vi "Host_AutoApproach.vi"() -> ()   [LabVIEW 2014]
uses:
  <vilib>/userdefined/High Color/nirio_resource_hc.ctl
  <vilib>/Instr/_visa.llb/VISA Configure Serial Port (Instr).vi
  <vilib>/FPGAPlugInAG/PCIe-7851R/niLvFpga_Open_PCIe-7851R.vi
  <vilib>/rvi/interface/common/dynamic/niFpgaDynamicAddResources.vi
  <vilib>/Utility/error.llb/Error Cluster From Error Code.vi
  <vilib>/rvi/errors/niLvFpgaAdjustHostInterfaceError.vi
  <vilib>/FPGAPlugInAG/Dynamic/niLvFpga_Run_Dynamic.vi
  <vilib>/FPGAPlugInAG/Dynamic/niLvFpga_Close_Dynamic.vi
  <vilib>/rvi/interface/nirviOpenFPGA/nirviOpenFPGA.xnode
  FPGA Bitfiles/XZFPGAWithinHopp_FPGATarget_ApproachingStep(_Flh4bpoPuwk.lvbitx
  <vilib>/rvi/interface/nirviReadWriteControl/nirviReadWriteControl.xnode
  <vilib>/rvi/interface/nirviMethod/nirviMethod.xnode
  <vilib>/rvi/interface/nirviCloseFPGA/nirviCloseFPGA.xnode
  NiFpgaLv.dll
  <vilib>/rvi/interface/Simulation/niFpgaSimulationCallBeginRW.vi
panel:
  out "ZCalPos":i32
  in  "PIZ":T1
  in  "ContinuousReapproach":bool
  in  "UseMemoryPos?":bool=TRUE
  out "ZRealPos":i16
  out "Curr":i16
  out "PIZPosDia":i16(graph)
  out "CurrDia":i16(graph)
  in  "stop":bool
  out "RoughZPos?":dbl
  out "Error?":string
  in  "RoughZ":refnum<visa-resource-name>
  in  "RoughZInitPos":dbl format="%#_13g"
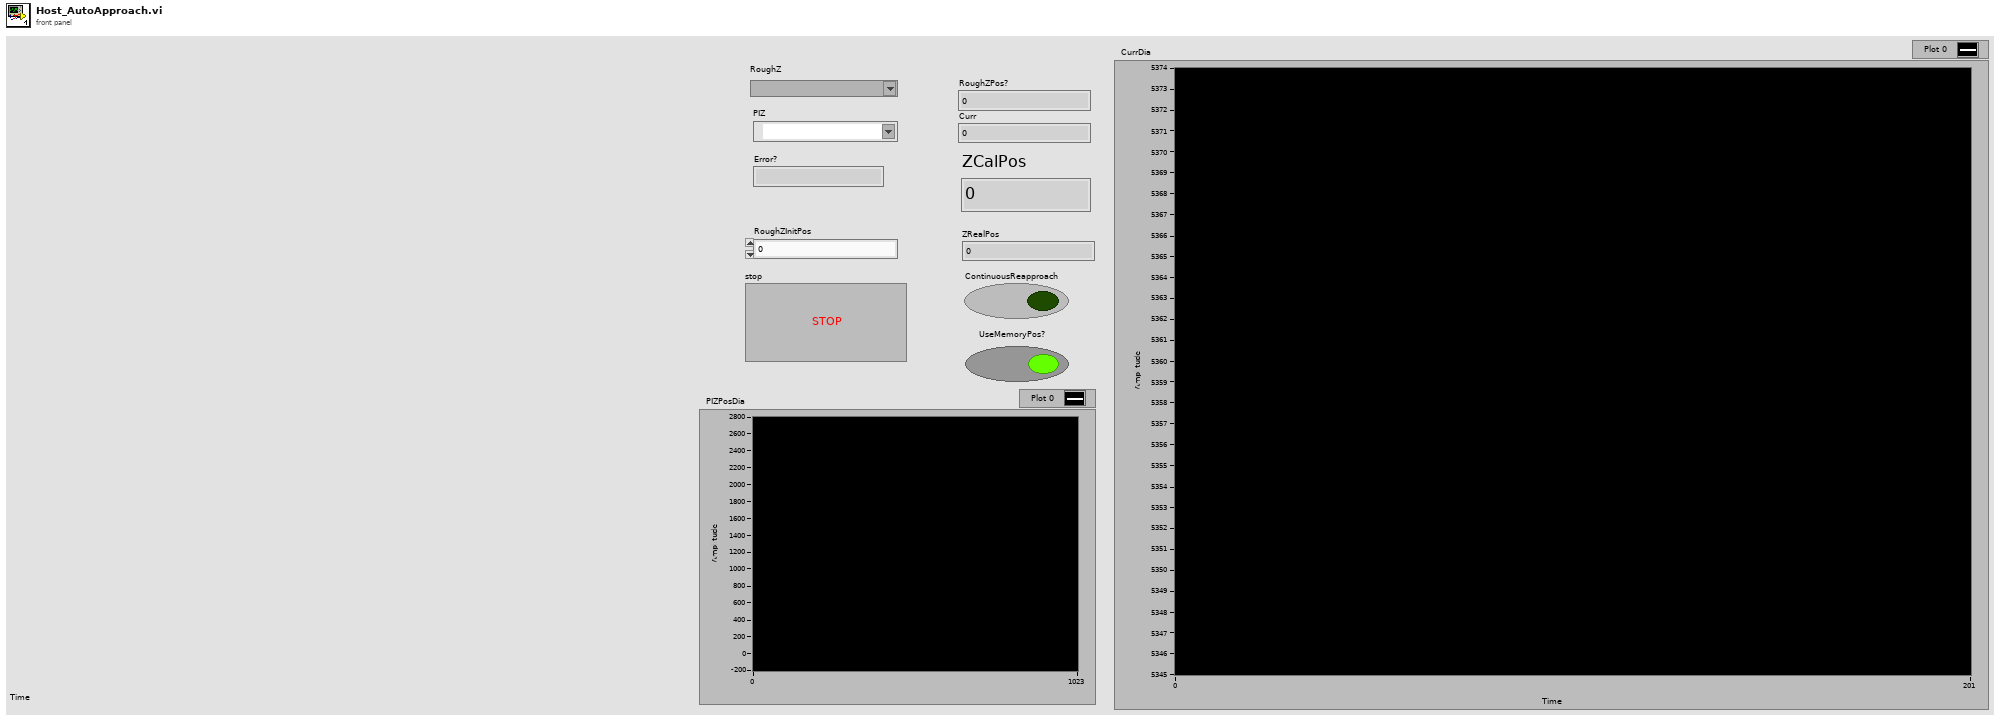
[diagram p1: front panel]
types:
  T1 = typedef "nirio_resource_hc.ctl" = tag
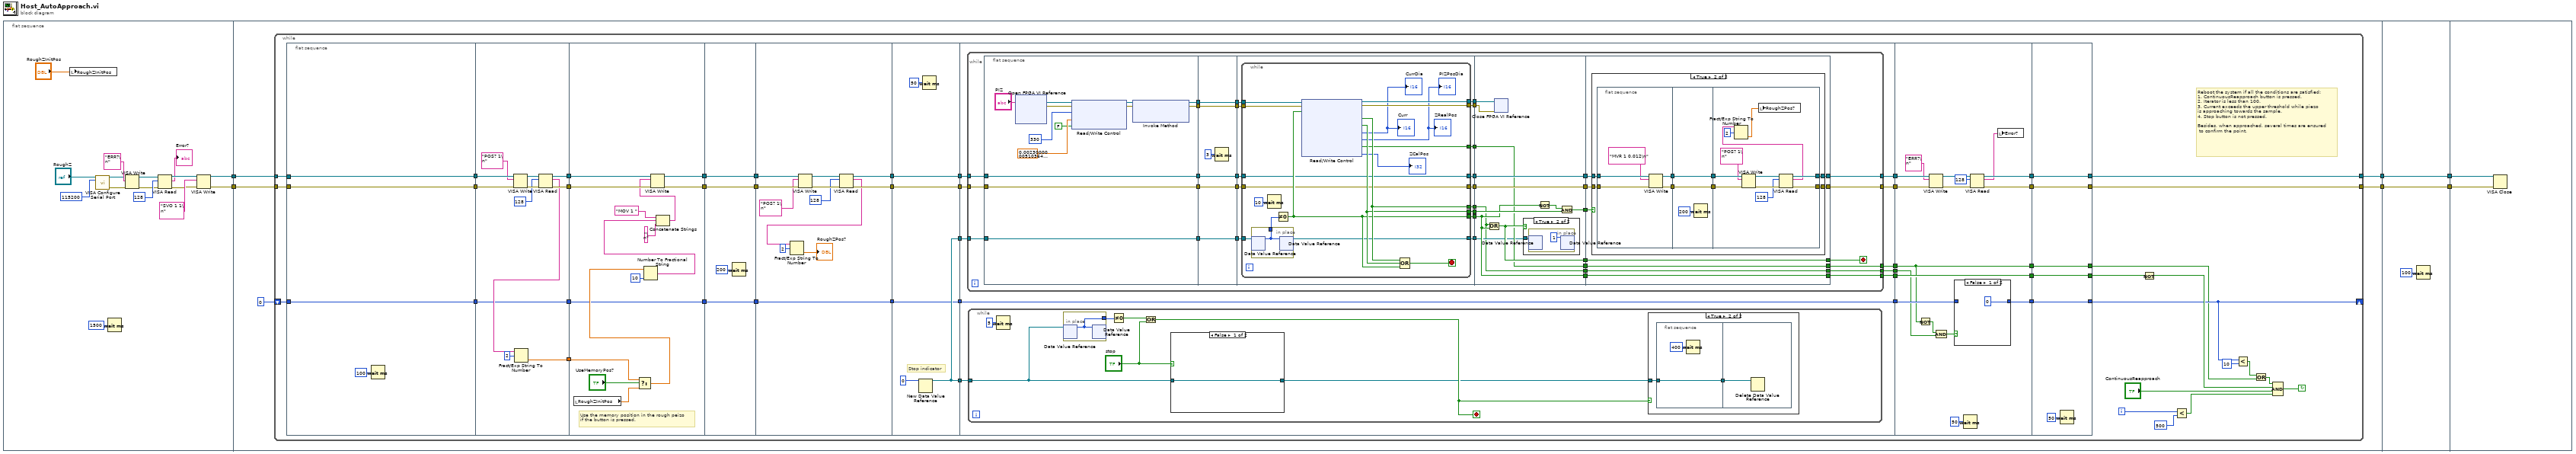
[diagram p0: block diagram]
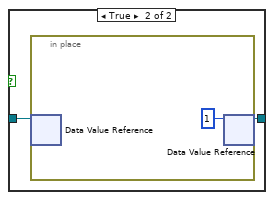
[diagram p3: hidden frame]
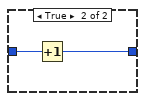
[diagram p6: hidden frame]
diagram:
  n1 = flat-sequence {
    tunnel: [w8] -> w2
    tunnel: [w7] -> w1
    tunnel: [w26] -> w5
    tunnel: [w25] -> w3
    tunnel: w2 -> [w24]
    tunnel: w1 -> [w23]
    tunnel: [w323] -> w6
    tunnel: w5 -> [w323]
    tunnel: [w322] -> w4
    tunnel: w3 -> [w322]
    tunnel: w6 -> [w325]
    tunnel: w4 -> [w324]
    frame #0 {
      n2 = local write "RoughZInitPos"("RoughZInitPos") -> ()
      n3 = call-poly "VISA Configure Serial Port"("VISA resource name"="RoughZ", "baud rate (9600)"=u32 115200) -> ("VISA resource name out"=w11:refnum<visa-resource-name>, "error out"=w12:errorcluster)  [unwired: 12 in]
      n4 = Wait (ms)(milliseconds to wait=u32 1500) -> ()  [unwired: 1 out]
      n5 = VISA Write(VISA resource name=w11, write buffer="ERR?\n", error in (no error)=w12) -> (VISA resource name out=w14:refnum<visa-resource-name>, error out=w15:errorcluster)  [unwired: 1 out]
      n6 = VISA Read(VISA resource name=w14, byte count=u32 128, error in (no error)=w15) -> (VISA resource name out=w18:refnum<visa-resource-name>, read buffer=→"Error?":string, error out=w19:errorcluster)  [unwired: 1 out]
      n7 = VISA Write(VISA resource name=w18, write buffer="SVO 1 1\n", error in (no error)=w19) -> (VISA resource name out=w8:refnum<visa-resource-name>, error out=w7:errorcluster)  [unwired: 1 out]
    }
    frame #1 {
      n8 = while {
        shift-right: [w36] -> _
        shift-left: 0 -> [w46]
        tunnel: [w31] -> w26
        tunnel: [w30] -> w25
        tunnel: w24 -> [w29]
        tunnel: w23 -> [w28]
        i -> [w57]
        stop <- w51 continue-if-true
        # "Reboot the system if all the conditions are satisfied:\n1. ContinuousReapproach button is pressed.\n2. Iterator is less than 100.\n3. Current exceeds the upper threshold while piezo\nis approaching towards the sample.\n4. Stop button is not pressed.\n\nBesides, when approached, several times are ensured\n to confirm the point."
        n9 = flat-sequence {
          tunnel: [w78] -> w76
          tunnel: [w77] -> w75
          tunnel: w46 -> [w80]
          tunnel: [w80] -> w45
          tunnel: w29 -> [w78]
          tunnel: w28 -> [w77]
          tunnel: w76 -> [w92]
          tunnel: [w88] -> w74
          tunnel: w75 -> [w91]
          tunnel: [w87] -> w73
          tunnel: [w82] -> w72
          tunnel: w45 -> [w81]
          tunnel: [w81] -> w44
          tunnel: w74 -> [w106]
          tunnel: w73 -> [w105]
          tunnel: [w99] -> w71
          tunnel: [w98] -> w70
          tunnel: w72 -> [w96]
          tunnel: w44 -> [w93]
          tunnel: [w93] -> w41
          tunnel: w71 -> [w110]
          tunnel: w70 -> [w109]
          tunnel: [w110] -> w69
          tunnel: [w109] -> w68
          tunnel: [w107] -> w42
          tunnel: w41 -> [w107]
          tunnel: w69 -> [w122]
          tunnel: w68 -> [w121]
          tunnel: [w116] -> w67
          tunnel: [w115] -> w66
          tunnel: [w111] -> w43
          tunnel: w42 -> [w111]
          tunnel: [w128] -> w65
          tunnel: [w127] -> w64
          tunnel: [w124] -> w63
          tunnel: [w124] -> w62
          tunnel: w66 -> [w127]
          tunnel: w67 -> [w128]
          tunnel: w43 -> [w123]
          tunnel: [w123] -> w40
          tunnel: w65 -> [w138]
          tunnel: w64 -> [w137]
          tunnel: w63 -> [w136]
          tunnel: w62 -> [w135]
          tunnel: [w134] -> w61
          tunnel: [w133] -> w60
          tunnel: [w132] -> w55
          tunnel: [w131] -> w50
          tunnel: w40 -> [w130]
          tunnel: [w130] -> w39
          tunnel: [w129] -> w38
          tunnel: w61 -> [w311]
          tunnel: w60 -> [w310]
          tunnel: [w305] -> w59
          tunnel: [w304] -> w58
          tunnel: w55 -> [w300]
          tunnel: [w300] -> w54
          tunnel: w50 -> [w297]
          tunnel: [w297] -> w49
          tunnel: w39 -> [w301]
          tunnel: w38 -> [w295]
          tunnel: [w298] -> w37
          tunnel: [w319] -> w48
          tunnel: [w318] -> w33
          tunnel: [w317] -> w31
          tunnel: [w316] -> w30
          tunnel: w49 -> [w318]
          tunnel: w54 -> [w319]
          tunnel: w58 -> [w316]
          tunnel: w59 -> [w317]
          tunnel: w37 -> [w315]
          tunnel: [w315] -> w36
          frame #0 {
            n10 = Wait (ms)(milliseconds to wait=u32 100) -> ()  [unwired: 1 out]
          }
          frame #1 {
            n11 = VISA Write(VISA resource name=w92, write buffer="POS? 1\n", error in (no error)=w91) -> (VISA resource name out=w90:refnum<visa-resource-name>, error out=w89:errorcluster)  [unwired: 1 out]
            n12 = VISA Read(VISA resource name=w90, byte count=u32 128, error in (no error)=w89) -> (VISA resource name out=w88:refnum<visa-resource-name>, read buffer=w84:string, error out=w87:errorcluster)  [unwired: 1 out]
            n13 = Fract/Exp String To Number(string=w84, offset=2) -> (number=w82:dbl)  [unwired: 2 in, 1 out]
          }
          frame #2 {
            # "Use the memory position in the rough peizo\nif the button is pressed."
            n14 = local read "RoughZInitPos"() -> (w95:dbl)
            n15 = Select(t=w96, s="UseMemoryPos?", f=w95) -> (s? t:f=w94:dbl)
            n16 = Number To Fractional String(number=w94, precision (6)=i16 10) -> (F-format string=w102:string)  [unwired: 2 in]
            n17 = Concatenate Strings("MOV 1 " ("string"), w102, "\n" ("string")) -> (w104:string)
            n18 = VISA Write(VISA resource name=w106, write buffer=w104, error in (no error)=w105) -> (VISA resource name out=w99:refnum<visa-resource-name>, error out=w98:errorcluster)  [unwired: 1 out]
          }
          frame #3 {
            n19 = Wait (ms)(milliseconds to wait=u32 200) -> ()  [unwired: 1 out]
          }
          frame #4 {
            n20 = VISA Write(VISA resource name=w122, write buffer="POS? 1\n", error in (no error)=w121) -> (VISA resource name out=w119:refnum<visa-resource-name>, error out=w118:errorcluster)  [unwired: 1 out]
            n21 = VISA Read(VISA resource name=w119, byte count=u32 128, error in (no error)=w118) -> (VISA resource name out=w116:refnum<visa-resource-name>, read buffer=w114:string, error out=w115:errorcluster)  [unwired: 1 out]
            n22 = Fract/Exp String To Number(string=w114, offset=2) -> (number=→"RoughZPos?":dbl)  [unwired: 2 in, 1 out]
          }
          frame #5 {
            # "Stop indicator"
            n23 = New Data Value Reference(data value=0) -> (data value reference=w124:refnum<data-value>)  [unwired: 1 in, 1 out]
            n24 = Wait (ms)(milliseconds to wait=u32 50) -> ()  [unwired: 1 out]
          }
          frame #6 {
            n25 = while {
              tunnel: w138 -> [w190]
              tunnel: w137 -> [w189]
              tunnel: w135 -> [w188]
              tunnel: [w174] -> w134
              tunnel: [w173] -> w133
              tunnel: [w171] -> w132
              tunnel: [w168] -> w131
              tunnel: [w156] -> w129
              stop <- w175 stop-if-true
              n26 = flat-sequence {
                tunnel: w190 -> [w200]
                tunnel: w189 -> [w199]
                tunnel: [w203] -> w167
                tunnel: [w202] -> w165
                tunnel: [w201] -> w163
                tunnel: w188 -> [w201]
                tunnel: [w200] -> w161
                tunnel: [w199] -> w159
                tunnel: w167 -> [w209]
                tunnel: [w209] -> w166
                tunnel: w165 -> [w208]
                tunnel: [w208] -> w164
                tunnel: w163 -> [w207]
                tunnel: [w207] -> w162
                tunnel: w161 -> [w206]
                tunnel: [w206] -> w160
                tunnel: w159 -> [w205]
                tunnel: [w205] -> w158
                tunnel: w166 -> [w223]
                tunnel: w164 -> [w222]
                tunnel: w162 -> [w221]
                tunnel: w160 -> [w220]
                tunnel: w158 -> [w219]
                tunnel: [w218] -> w187
                tunnel: [w217] -> w186
                tunnel: [w216] -> w185
                tunnel: [w215] -> w184
                tunnel: [w214] -> w183
                tunnel: [w213] -> w182
                tunnel: [w212] -> w181
                tunnel: [w211] -> w180
                tunnel: [w210] -> w170
                tunnel: w187 -> [w243]
                tunnel: w186 -> [w251]
                tunnel: w185 -> [w246]
                tunnel: w184 -> [w254]
                tunnel: w183 -> [w253]
                tunnel: w182 -> [w248]
                tunnel: w181 -> [w249]
                tunnel: w180 -> [w244]
                tunnel: [w250] -> w179
                tunnel: [w249] -> w178
                tunnel: [w248] -> w177
                tunnel: [w247] -> w176
                tunnel: [w246] -> w172
                tunnel: w170 -> [w245]
                tunnel: [w245] -> w169
                tunnel: [w243] -> w157
                tunnel: w179 -> [w265]
                tunnel: w178 -> [w264]
                tunnel: w177 -> [w263]
                tunnel: w176 -> [w262]
                tunnel: [w262] -> w175
                tunnel: [w261] -> w174
                tunnel: [w260] -> w173
                tunnel: w172 -> [w259]
                tunnel: [w259] -> w171
                tunnel: w169 -> [w258]
                tunnel: [w258] -> w168
                tunnel: w157 -> [w257]
                tunnel: [w257] -> w156
                frame #0 {
                  n27 = xnode "Open FPGA VI Reference"("resource name"="PIZ") -> ("FPGA VI Reference Out"=w197:refnum<k20>, "error out"=w195:errorcluster)  [unwired: 1 in]
                  n28 = xnode "Read/Write Control"("FPGA VI Reference In"=w197, "error in"=w195, "Count(uSec)"=u32 330, "Threshold"=sgl 0.0023, "DefaultThreshold?"=FALSE) -> ("FPGA VI Reference Out"=w196:refnum<k20>, "error out"=w194:errorcluster)
                  n29 = xnode "Invoke Method"("FPGA VI Reference In"=w196, "error in"=w194) -> ("FPGA VI Reference Out"=w203:refnum<k20>, "error out"=w202:errorcluster)  [unwired: 1 in]
                }
                frame #1 {
                  n30 = Wait (ms)(milliseconds to wait=u32 3) -> ()  [unwired: 1 out]
                }
                frame #2 {
                  n31 = while {
                    tunnel: w223 -> [w241]
                    tunnel: w222 -> [w240]
                    tunnel: w221 -> [w239]
                    tunnel: w220 -> [w231]
                    tunnel: w219 -> [w230]
                    tunnel: [w236] -> w218
                    tunnel: [w235] -> w217
                    tunnel: [w234] -> w216
                    tunnel: [w233] -> w215
                    tunnel: [w232] -> w214
                    tunnel: [w231] -> w212
                    tunnel: [w230] -> w213
                    tunnel: [w229] -> w211
                    tunnel: [w226] -> w210
                    stop <- w237 stop-if-true
                    n32 = in-place {
                      in-place-border: [w242] -> w238
                      n33 = in-place-dvr #1(w239) -> (w242:i32)  [unwired: 1 out]
                      n34 = in-place-dvr #1(w242) -> (w229:refnum<data-value>)  [unwired: 1 out]
                    }
                    n35 = Wait (ms)(milliseconds to wait=u32 10) -> ()  [unwired: 1 out]
                    n36 = Not Equal To 0?(x=w238) -> (x != 0?=w234:bool)
                    n37 = xnode "Read/Write Control"("FPGA VI Reference In"=w241, "error in"=w240, "stop"=w234) -> ("FPGA VI Reference Out"=w233:refnum<k20>, "error out"=w232:errorcluster, "Approached?"=w236:bool, "PIZRangeExceeded?"=w235:bool, "PresCurr"=→"CurrDia" →"Curr":i16, "RealPIZPos"=→"PIZPosDia" →"ZRealPos":i16, "ExceedUpperLimit?"=w226:bool, "ZCalPos"=→"ZCalPos":i32)
                    n38 = Compound Arithmetic op=OR(w236, w235, w234) -> (w237:bool)
                  }
                }
                frame #3 {
                  n39 = Or(x=w243, y=w246) -> (x .or. y?=w247:bool)
                  n40 = xnode "Close FPGA VI Reference"("FPGA VI Reference In"=w254, "error in"=w253) -> ()  [unwired: 1 out]
                  n41 = case shown="True" w247 {
                    tunnel: w244 -> [_ w255]
                    frame False {
                    }
                    frame True {
                      n42 = in-place {
                        n43 = in-place-dvr #2(w255) -> ()  [unwired: 2 out]
                        n44 = in-place-dvr #2(1 ("data value")) -> ()  [unwired: 2 out]
                      }
                    }
                  }
                  n45 = Not(x=w246) -> (.not. x?=w252:bool)
                  n46 = And(x=w252, y=w251) -> (x .and. y?=w250:bool)
                }
                frame #4 {
                  n47 = case shown="True" w265 {
                    tunnel: w264 -> [w267 w275]
                    tunnel: w263 -> [w266 w274]
                    tunnel: [w267 w269] -> w261
                    tunnel: [w266 w268] -> w260
                    frame False {
                    }
                    frame True {
                      n48 = flat-sequence {
                        tunnel: w275 -> [w280]
                        tunnel: w274 -> [w279]
                        tunnel: [w277] -> w273
                        tunnel: [w276] -> w272
                        tunnel: w273 -> [w283]
                        tunnel: w272 -> [w282]
                        tunnel: [w283] -> w271
                        tunnel: [w282] -> w270
                        tunnel: w271 -> [w294]
                        tunnel: w270 -> [w293]
                        tunnel: [w288] -> w269
                        tunnel: [w287] -> w268
                        frame #0 {
                          n49 = VISA Write(VISA resource name=w280, write buffer="MVR 1 0.012\n", error in (no error)=w279) -> (VISA resource name out=w277:refnum<visa-resource-name>, error out=w276:errorcluster)  [unwired: 1 out]
                        }
                        frame #1 {
                          n50 = Wait (ms)(milliseconds to wait=u32 200) -> ()  [unwired: 1 out]
                        }
                        frame #2 {
                          n51 = VISA Write(VISA resource name=w294, write buffer="POS? 1\n", error in (no error)=w293) -> (VISA resource name out=w291:refnum<visa-resource-name>, error out=w290:errorcluster)  [unwired: 1 out]
                          n52 = VISA Read(VISA resource name=w291, byte count=u32 128, error in (no error)=w290) -> (VISA resource name out=w288:refnum<visa-resource-name>, read buffer=w286:string, error out=w287:errorcluster)  [unwired: 1 out]
                          n53 = Fract/Exp String To Number(string=w286, offset=2) -> (number=w284:dbl)  [unwired: 2 in, 1 out]
                          n54 = local write "RoughZPos?"(w284) -> ()
                        }
                      }
                    }
                  }
                }
              }
            }
            n55 = while {
              tunnel: w136 -> [w144]
              stop <- w140 stop-if-true
              n56 = Wait (ms)(milliseconds to wait=u32 5) -> ()  [unwired: 1 out]
              n57 = in-place {
                in-place-border: [w151] -> w143
                n58 = in-place-dvr #3(w144) -> (w151:i32)  [unwired: 1 out]
                n59 = in-place-dvr #3(w151) -> ()  [unwired: 2 out]
              }
              n60 = Not Equal To 0?(x=w143) -> (x != 0?=w142:bool)
              n61 = Or(x=w142, y="stop") -> (x .or. y?=w140:bool)
              n62 = case shown="False" "stop" {
                tunnel: w144 -> [w152 w154]
                tunnel: [w152 w153] -> w139
                frame False {
                }
                frame True {
                  n63 = in-place {
                    n64 = in-place-dvr #4(w154) -> ()  [unwired: 2 out]
                    n65 = in-place-dvr #4(1 ("data value")) -> (w153:refnum<data-value>)  [unwired: 1 out]
                  }
                }
              }
              n66 = case shown="True" w140 {
                tunnel: w139 -> [_ w147]
                frame False {
                }
                frame True {
                  n67 = flat-sequence {
                    tunnel: w147 -> [w148]
                    tunnel: [w148] -> w146
                    tunnel: w146 -> [w150]
                    frame #0 {
                      n68 = Wait (ms)(milliseconds to wait=u32 400) -> ()  [unwired: 1 out]
                    }
                    frame #1 {
                      n69 = Delete Data Value Reference(data value reference=w150) -> ()  [unwired: 1 in, 2 out]
                    }
                  }
                }
              }
            }
          }
          frame #7 {
            n70 = Not(x=w297) -> (.not. x?=w296:bool)
            n71 = VISA Write(VISA resource name=w311, write buffer="ERR?\n", error in (no error)=w310) -> (VISA resource name out=w309:refnum<visa-resource-name>, error out=w308:errorcluster)  [unwired: 1 out]
            n72 = Compound Arithmetic op=AND(w296, w295) -> (w299:bool)
            n73 = case shown="False" w299 {
              tunnel: w301 -> [_ w314]
              tunnel: [0 w313] -> w298
              frame False {
              }
              frame True {
                n74 = Increment(x=w314) -> (x+1=w313:i32)
              }
            }
            n75 = Wait (ms)(milliseconds to wait=u32 50) -> ()  [unwired: 1 out]
            n76 = VISA Read(VISA resource name=w309, byte count=u32 128, error in (no error)=w308) -> (VISA resource name out=w305:refnum<visa-resource-name>, read buffer=w303:string, error out=w304:errorcluster)  [unwired: 1 out]
            n77 = local write "Error?"(w303) -> ()
          }
          frame #8 {
            n78 = Wait (ms)(milliseconds to wait=u32 50) -> ()  [unwired: 1 out]
          }
        }
        n79 = Not(x=w48) -> (.not. x?=w47:bool)
        n80 = Less?(x=w57, y=500) -> (x < y?=w52:bool)
        n81 = Less?(x=w36, y=10) -> (x < y?=w34:bool)
        n82 = Or(x=w34, y=w33) -> (x .or. y?=w32:bool)
        n83 = Compound Arithmetic op=AND(w32, w47, "ContinuousReapproach", w52) -> (w51:bool)
      }
    }
    frame #2 {
      n84 = Wait (ms)(milliseconds to wait=u32 100) -> ()  [unwired: 1 out]
    }
    frame #3 {
      n85 = VISA Close(VISA resource name=w325, error in (no error)=w324) -> ()  [unwired: 1 out]
    }
  }
